vi "Load Modules.vi"(0 "Configuration folder":path, 7 "Modules folder":path, 9 "Open Frontpanel (VI Namei)":string[](array[string]), 11 "error in (no error)":errorcluster) -> (4 "VI Refs Out":refnum<vi>[](array[refnum]), 8 "Found VI":string[](array[string]), 15 "error out":errorcluster)   [LabVIEW 2019, in "Subpanel Tools.lvlib"]
doc: "This VI loads other VI by VI Server."
uses:
  Subpanel Tools.lvlib
  Message Queue/State Name.ctl
  Global - Name of loaded Module.vi
  Message Queue/Message Queue.lvlib
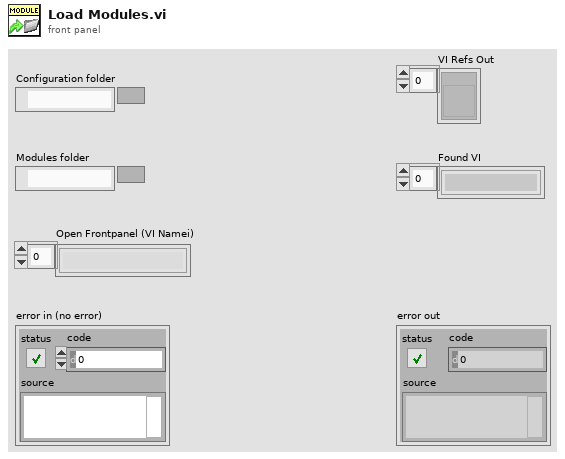
[diagram p1: front panel]
types:
  T1 = typedef "Message Queue.lvlib/State Name.ctl" = enum16{"Default", "Initialize", "Initialize Data", "Initialize Modules", "Initialize Panel", "Close FP", "Open FP", "Initialize Menu", "Mode", "Update Subpanel", "Error", "Open Help", "About", "Open WebResources", "Exit"}
  T2 = enum16{"open", "replace", "create", "open or create", "replace or create", "replace or create with confirmation"}
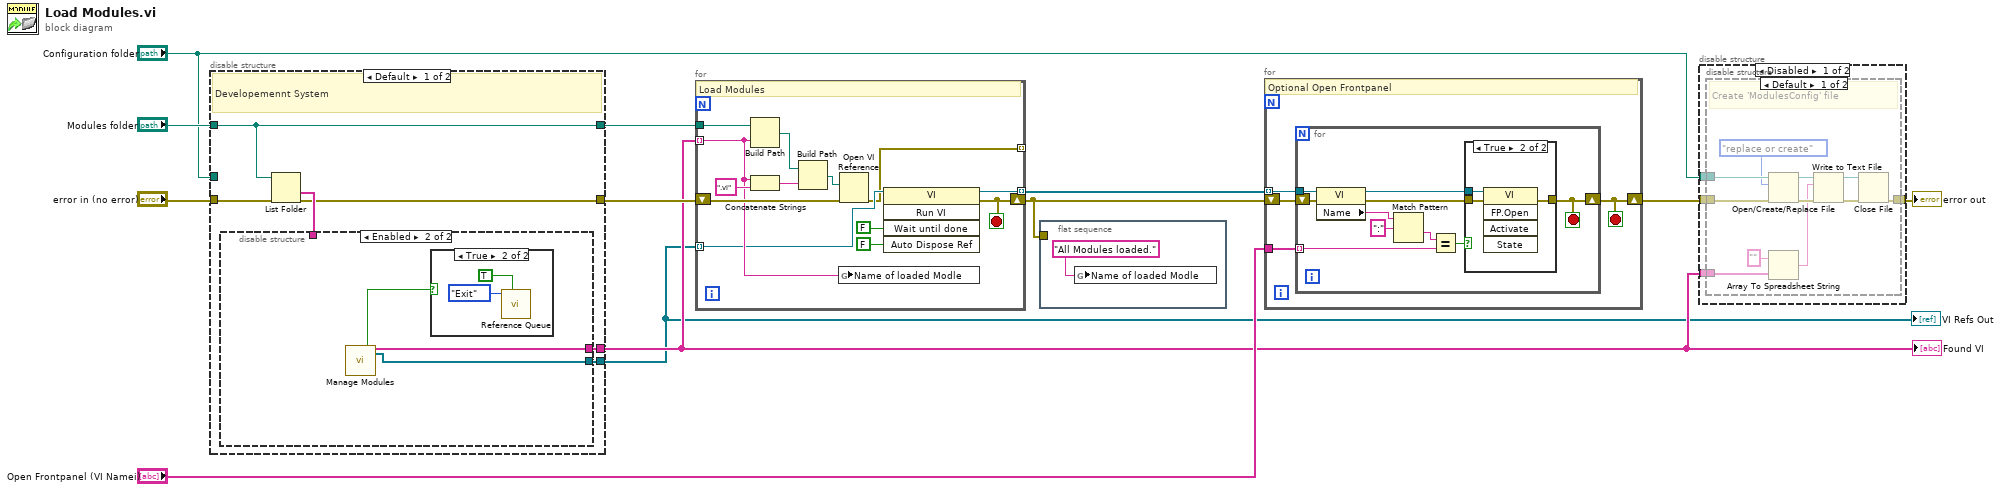
[diagram p0: block diagram]
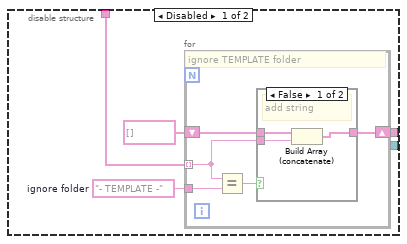
[diagram p4: hidden frame]
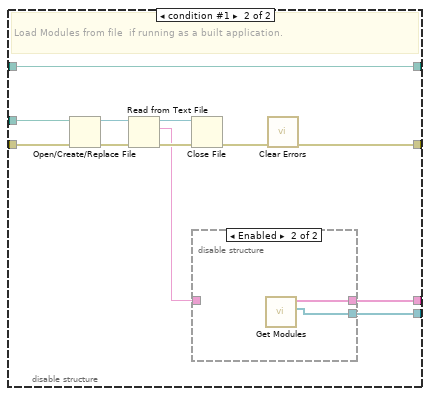
[diagram p7: hidden frame]
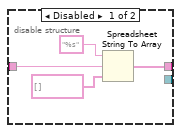
[diagram p8: hidden frame]
diagram:
  n1 = disable-structure shown="Default" {
    disable-tunnel: [w17 w42] -> w5
    disable-tunnel: [w15 w38] -> w7
    disable-tunnel: "error in (no error)" -> [w16 w44]
    disable-tunnel: "Modules folder" -> [w14 w40]
    disable-tunnel: [w14 w40] -> w6
    disable-tunnel: "Configuration folder" -> [_ w43]
    disable-tunnel: [w13 w37] -> w1
    frame condition #0 (active) {
      # "Developemennt System"
      n2 = List Folder(path=w14, error in=w16) -> (folder names=w18:string[], error out=w15:errorcluster)  [unwired: 2 in, 2 out]
      n3 = disable-structure shown="Enabled" {
        disable-tunnel: w18 -> [w22 _]
        disable-tunnel: [w19 w34] -> w17
        disable-tunnel: [_ w33] -> w13
        frame Disabled {
          w20 = "- TEMPLATE -"  # ignore folder
          n4 = for {
            tunnel: w22 -> [w24] mode=indexing
            shift-right: [w26] -> w19
            shift-left: string[] [] -> [w27]
            tunnel: w20 -> [w25]
            # "ignore TEMPLATE folder"
            n5 = Equal?(x=w24, y=w25) -> (x = y?=w23:bool)
            n6 = case shown="False" w23 {
              tunnel: w27 -> [w30 w31]
              tunnel: [w29 w31] -> w26
              tunnel: w24 -> [w28 _]
              frame False {
                # "add string"
                n7 = Build Array (concatenate)(w30, w28) -> (w29:string[])
              }
              frame True {
                # "ignore string"
              }
            }
          }
        }
        frame Enabled {
          n8 = call "Manage Modules.vi"() -> ("Cancelled?"=w32:bool, "Selected Modules"=w34:string[], "Modules Refs"=w33:refnum<vi>[])  [unwired: 17 in]
          n9 = case shown="True" w32 {
            frame False {
            }
            frame True {
              n10 = call "Reference Queue.vi"("Priority Message? (F)"=TRUE, "Tasks"=State_Name."Exit") -> ()  [unwired: 9 in, 1 out]
            }
          }
        }
      }
    }
    frame condition #1 {
      # "Load Modules from file  if running as a built application."
      n11 = Open/Create/Replace File(file path (use dialog)=w43, error in=w44) -> (refnum out=w46:refnum<file>, error out=w48:errorcluster)  [unwired: 4 in, 1 out]
      n12 = Read from Text File(file (use dialog)=w46, error in=w48) -> (refnum out=w45:refnum<file>, text=w41:string, error out=w47:errorcluster)  [unwired: 2 in, 1 out]
      n13 = Close File(refnum=w45, error in=w47) -> (error out=w39:errorcluster)  [unwired: 1 out]
      n14 = disable-structure shown="Enabled" {
        disable-tunnel: [w52 w54] -> w42
        disable-tunnel: w41 -> [w51 _]
        disable-tunnel: [_ w53] -> w37
        frame Disabled {
          n15 = Spreadsheet String To Array(format string="%s", spreadsheet string=w51, array type (2D Dbl)=string[] []) -> (array=w52:string[])  [unwired: 1 in]
        }
        frame Enabled {
          n16 = call "Get Modules.vi"() -> ("Modules Refs"=w53:refnum<vi>[], "Modules Names"=w54:string[])  [unwired: 8 in, 2 out]
        }
      }
      n17 = call <vilib>:"Clear Errors.vi"("error in (no error)"=w39) -> ("error out"=w38:errorcluster)  [unwired: 5 in, 1 out]
    }
  }
  "VI Refs Out" <- w1
  "Found VI" <- w5
  n18 = for {
    tunnel: w6 -> [w63]
    tunnel: w5 -> [w57] mode=indexing
    shift-right: [w61] -> w2
    shift-left: w7 -> [w67]
    tunnel: [w62] -> w11 mode=indexing
    tunnel: w1 -> [w56] mode=indexing
    tunnel: [w55] -> _ mode=indexing
    stop <- w61 stop-if-true
    # "Load Modules"
    n19 = Build Path(base path=w63, name or relative path=w57) -> (appended path=w60:path)
    n20 = Concatenate Strings(w57, ".vi" ("String")) -> (w58:string)
    n21 = Build Path(base path=w60, name or relative path=w58) -> (appended path=w59:path)
    n22 = global write "Global - Name of loaded Module.vi" "Name of loaded Modle"(w57) -> ()
    n23 = Open VI Reference(vi path=w59, error in (no error)=w67) -> (error out=w55:errorcluster)  [unwired: 4 in, 1 out]
    n24 = invoke class="VI" method="Run VI"(reference=w56, "Wait until done"=FALSE ("Wait Until Done"), "Auto Dispose Ref"=FALSE ("Auto Dispose Reference")) -> (reference out=w62:refnum<vi>, error out=w61:errorcluster)  [unwired: 2 in, 3 out]
  }
  n25 = flat-sequence {
    tunnel: w2 -> [_]
    frame #0 {
      n26 = global write "Global - Name of loaded Module.vi" "Name of loaded Modle"("All Modules loaded.") -> ()
    }
  }
  n27 = for {
    shift-right: [w70] -> w9
    shift-left: w2 -> [w72]
    tunnel: w11 -> [w71] mode=indexing
    tunnel: "Open Frontpanel (VI Namei)" -> [w69]
    stop <- w70 stop-if-true
    # "Optional Open Frontpanel"
    n28 = for {
      tunnel: w71 -> [w81]
      shift-right: [w82] -> w70
      shift-left: w72 -> [w80]
      tunnel: w69 -> [w77] mode=indexing
      stop <- w82 stop-if-true
      n29 = property class="VI"(reference=w81, error in=w80) -> (reference out=w79:refnum<vi>, error out=w78:errorcluster, "Name"=w75:string)
      n30 = Match Pattern(string=w75, regular expression=":") -> (after substring=w73:string)  [unwired: 1 in, 3 out]
      n31 = Equal?(x=w73, y=w77) -> (x = y?=w76:bool)
      n32 = case shown="True" w76 {
        tunnel: w79 -> [_ w86]
        tunnel: w78 -> [w83 w85]
        tunnel: [w83 w84] -> w82
        frame False {
        }
        frame True {
          n33 = invoke class="VI" method="FP.Open"(reference=w86, error in=w85) -> (error out=w84:errorcluster)  [unwired: 3 in, 4 out]
        }
      }
    }
  }
  n34 = disable-structure shown="Disabled" {
    disable-tunnel: w9 -> [w90 _]
    disable-tunnel: [w89 _] -> w8
    disable-tunnel: w5 -> [w88 _]
    disable-tunnel: "Configuration folder" -> [w87 _]
    frame Disabled {
      n35 = disable-structure shown="Default" {
        disable-tunnel: w90 -> [w101 w102]
        disable-tunnel: [w100 w102] -> w89
        disable-tunnel: w87 -> [w99 _]
        disable-tunnel: w88 -> [w98 _]
        frame condition #0 (active) {
          # "Create 'ModulesConfig' file"
          n36 = Open/Create/Replace File(file path (use dialog)=w99, error in=w101, operation (0:open)=T2."replace or create") -> (refnum out=w96:refnum<file>, error out=w97:errorcluster)  [unwired: 3 in, 1 out]
          n37 = Array To Spreadsheet String(array=w98, 3:"" ("format string")) -> (spreadsheet string=w93:string)  [unwired: 1 in]
          n38 = Write to Text File(file (use dialog)=w96, text=w93, error in=w97) -> (refnum out=w95:refnum<file>, error out=w94:errorcluster)  [unwired: 1 in, 1 out]
          n39 = Close File(refnum=w95, error in=w94) -> (error out=w100:errorcluster)  [unwired: 1 out]
        }
        frame condition #1 {
        }
      }
    }
    frame Enabled {
    }
  }
  "error out" <- w8
